vi "Write No Delay.vi"(8 "error in (no error)":errorcluster, 10 "No Delay":bool=TRUE, 11 "TCP Stream in":refnum<class "TCP Stream.lvclass">) -> (0 "error out":errorcluster, 3 "TCP Stream out":refnum<class "TCP Stream.lvclass">)   [LabVIEW 2020, in "TCP Stream.lvclass"]
uses:
  TCP Stream.lvclass
  TCP Stream.lvclass/TCP Stream.ctl
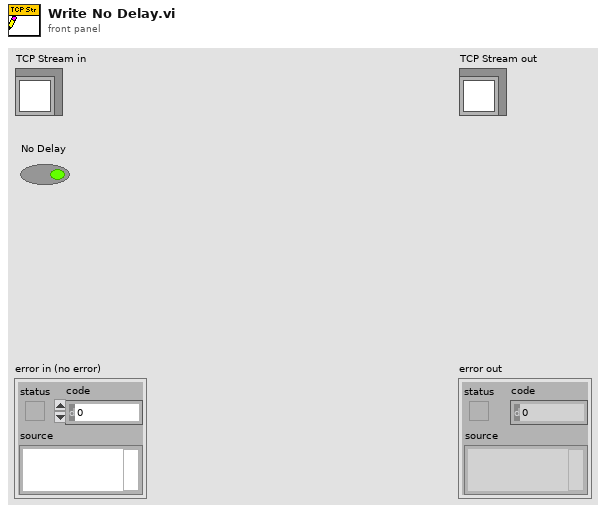
[diagram p1: front panel]
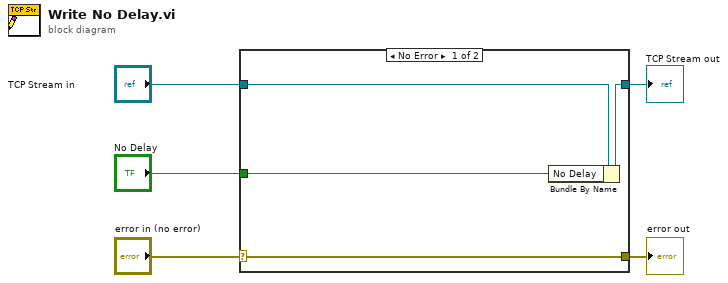
[diagram p0: block diagram]
diagram:
  n1 = case shown="No Error" "error in (no error)" {
    selector: "error in (no error)" -> [w9 w10]
    tunnel: [w9 w10] -> w4
    tunnel: [w7 w11] -> w2
    tunnel: "TCP Stream in" -> [w8 w11]
    tunnel: "No Delay" -> [w6 _]
    frame No Error {
      n2 = Bundle By Name(cluster=w8, "No Delay"=w6) -> (w7:refnum<class "TCP Stream.lvclass">)
    }
    frame Error {
    }
  }
  "error out" <- w4
  "TCP Stream out" <- w2
